vi "RTD_config_4wR.vi"(6 "range [Ohm]":dbl, 7 "type":T1=enum."COMET Tx5xx (ethernet)" caption="Type", 8 "error in":errorcluster, 11 "VISA in":refnum<visa-resource-name>) -> (0 "error out":errorcluster, 3 "VISA out":refnum<visa-resource-name>)   [LabVIEW 2020]
uses:
  thermo_types.ctl
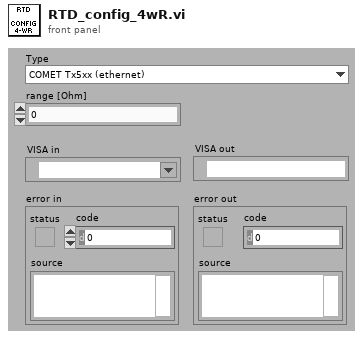
[diagram p1: front panel]
types:
  T1 = typedef "thermo_types.ctl" = enum16{"Disabled", "Simulated", "COMET Tx5xx (ethernet)", "Keithley 2002 (GPIB) + RTD", "Agilent 344xx (GPIB) + RTD"}
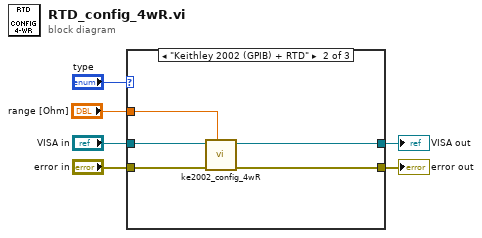
[diagram p0: block diagram]
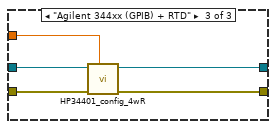
[diagram p3: hidden frame]
diagram:
  n1 = case shown="\"Keithley 2002 (GPIB) + RTD\"" "type" {
    tunnel: "error in" -> [w8 w13 w18]
    tunnel: [w8 w12 w17] -> w4
    tunnel: [w7 w11 w16] -> w3
    tunnel: "VISA in" -> [w7 w10 w15]
    tunnel: "range [Ohm]" -> [_ w9 w14]
    frame Default {
    }
    frame "Keithley 2002 (GPIB) + RTD" {
      n2 = call "ke2002_config_4wR.vi"("range value (ohms)"=w9, "error in"=w13, "VISA in"=w10) -> ("error out"=w12:errorcluster, "VISA out"=w11:refnum<visa-resource-name>)  [unwired: 7 in]
    }
    frame "Agilent 344xx (GPIB) + RTD" {
      n3 = call "HP34401_config_4wR.vi"("Manual Range (1.00)"=w14, "error in"=w18, "VISA in"=w15) -> ("error out"=w17:errorcluster, "VISA out"=w16:refnum<visa-resource-name>)  [unwired: 7 in]
    }
  }
  "error out" <- w4
  "VISA out" <- w3
